vi "only keep corners.vi"(11 "intensity values":dbl[][](array[numeric])) -> (3 "Array":i32[][](array[numeric]))   [LabVIEW 2016]
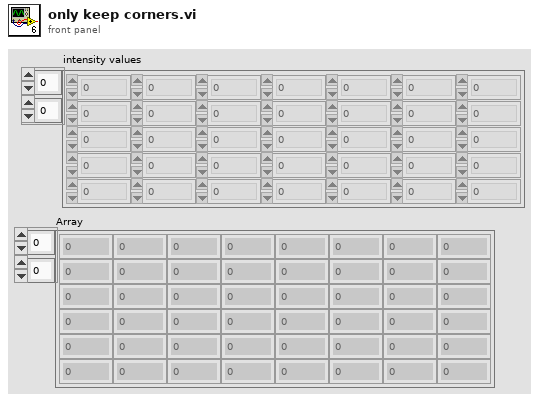
[diagram p1: front panel]
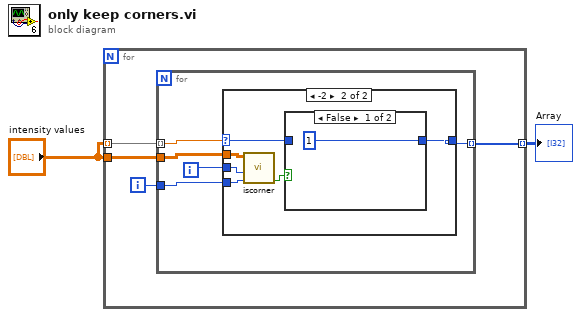
[diagram p0: block diagram]
diagram:
  n1 = for {
    tunnel: "intensity values" -> [w6] mode=indexing
    tunnel: "intensity values" -> [w5]
    tunnel: [w4] -> w1 mode=indexing
    i -> [w3]
    n2 = for {
      tunnel: w6 -> [w11] mode=indexing
      tunnel: w5 -> [w9]
      tunnel: [w10] -> w4 mode=indexing
      tunnel: w3 -> [w8]
      i -> [w7]
      n3 = case shown="-2" w11 {
        selector: w11 -> [w12 w18]
        tunnel: [w12 w17] -> w10
        tunnel: w9 -> [_ w16]
        tunnel: w8 -> [_ w14]
        tunnel: w7 -> [_ w15]
        frame 0, Default {
        }
        frame -2 {
          n4 = call "iscorner.vi"("index2"=w14, "index1"=w15, "intensity values"=w16) -> ("isCorner"=w13:bool)  [unwired: 8 in]
          n5 = case shown="False" w13 {
            tunnel: w18 -> [_ w20]
            tunnel: [1 w20] -> w17
            frame False {
            }
            frame True {
            }
          }
        }
      }
    }
  }
  "Array" <- w1
